vi "Four Flipping Coins.vi"() -> ()   [LabVIEW 2015]
uses:
  <vilib>/Analysis/NI_AALBase.lvlib
panel:
  out "Waveform Graph":i32[](graph)
  in  "# of Trials":dbl
  out "# of Heads":dbl
  out "Coin 4":bool
  out "Coin 3":bool
  out "Coin 2":bool
  out "Coin 1":bool
  # "Heads=Lit"
  # "Tails=Unlit"
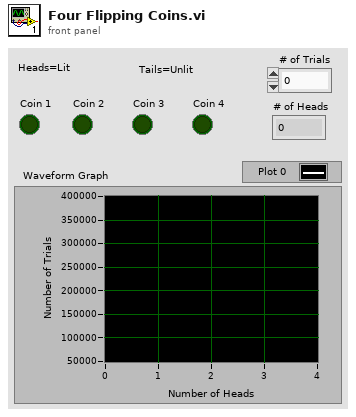
[diagram p1: front panel]
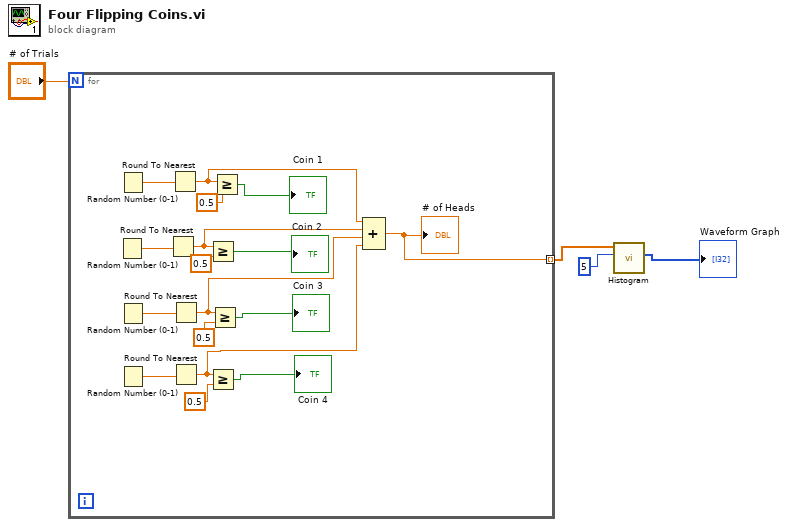
[diagram p0: block diagram]
diagram:
  n1 = for {
    N: "# of Trials" -> [_]
    tunnel: [w5] -> w3 mode=indexing
    n2 = Random Number (0-1)() -> (number: 0 to 1=w8:dbl)
    n3 = Random Number (0-1)() -> (number: 0 to 1=w9:dbl)
    n4 = Random Number (0-1)() -> (number: 0 to 1=w7:dbl)
    n5 = Random Number (0-1)() -> (number: 0 to 1=w6:dbl)
    n6 = Round To Nearest(number=w8) -> (nearest integer value=w12:dbl)
    n7 = Round To Nearest(number=w9) -> (nearest integer value=w13:dbl)
    n8 = Round To Nearest(number=w7) -> (nearest integer value=w11:dbl)
    n9 = Round To Nearest(number=w6) -> (nearest integer value=w10:dbl)
    n10 = Greater Or Equal?(x=w12, y=0.5) -> (x >= y?=→"Coin 2":bool)
    n11 = Greater Or Equal?(x=w10, y=0.5) -> (x >= y?=→"Coin 4":bool)
    n12 = Greater Or Equal?(x=w11, y=0.5) -> (x >= y?=→"Coin 3":bool)
    n13 = Greater Or Equal?(x=w13, y=0.5) -> (x >= y?=→"Coin 1":bool)
    n14 = Compound Arithmetic op=ADD(w13, w12, w11, w10) -> (w5:dbl)
    "# of Heads" <- w5
  }
  n15 = call <vilib>:"Histogram.vi"("intervals"=5, "X"=w3) -> ("Histogram: h(x)"=→"Waveform Graph":i32[])  [unwired: 6 in, 3 out]
